vi "Write Decorate.vi"(8 "error in":errorcluster, 10 "Decorate":refnum<class "Namer.lvclass">, 11 "Namer Decorator in":refnum<class "Namer Decorator.lvclass">) -> (0 "error out":errorcluster, 3 "Namer Decorator out":refnum<class "Namer Decorator.lvclass">)   [LabVIEW 2020, in "Approval Tests.lvlib" / "Namer Decorator.lvclass"]
uses:
  Namer Decorator.lvclass
  Namer/Namer.lvclass
  Namer Decorator.lvclass/Namer Decorator.ctl
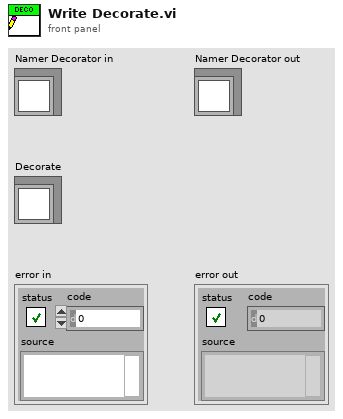
[diagram p1: front panel]
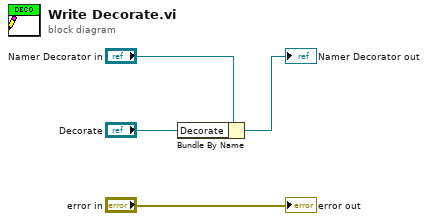
[diagram p0: block diagram]
diagram:
  n1 = Bundle By Name(cluster="Namer Decorator in", "Decorate"="Decorate") -> (→"Namer Decorator out":refnum<class "Namer Decorator.lvclass">)
  "error out" <- "error in"
